vi "OpenDBEditor.vi"   [LabVIEW 2021]
types:
  T1 = enum32{"Invalid", "Standard", "Closed", "Hidden", "Minimized", "Maximized"}
  T2 = typedef "ConfigurationData.ctl" = cluster{"DataSetFilePath":path, "DefaultErrorCreationType":string, "StartOfErrorRange":i32, "EndOfErrorRange":i32}
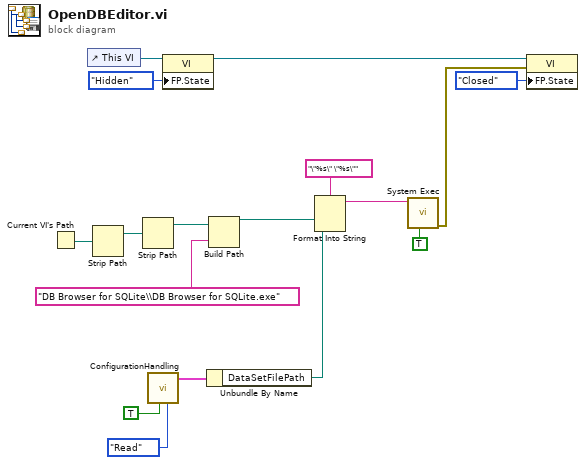
[diagram p0: block diagram]
diagram:
  n1 = Current VI's Path() -> (path=w16:path)
  n2 = control-ref of="This VI"() -> (w4:refnum<vi>)
  n3 = Strip Path(path=w16) -> (stripped path=w15:path)  [unwired: 1 out]
  n4 = Strip Path(path=w15) -> (stripped path=w14:path)  [unwired: 1 out]
  n5 = call "ConfigurationHandling.vi"("Function"=enum16{"Read", "Write"}."Read", "ForceReload"=TRUE) -> ("SettingsOut"=w8:T2)  [unwired: 9 in]
  n6 = property class="VI"(reference=w4, "FP.State"=T1."Hidden" ("Front Panel Window:State")) -> (reference out=w2:refnum<vi>)  [unwired: 1 in, 1 out]
  n7 = Unbundle By Name(w8) -> ("DataSetFilePath"=w7:path)
  n8 = Build Path(base path=w14, name or relative path="DB Browser for SQLite\\DB Browser for SQLite.exe") -> (appended path=w11:path)
  n9 = Format Into String(format string="\"%s\" \"%s\"" ("command line"), w11, w7) -> (resulting string=w6:string)  [unwired: 2 in, 1 out]
  n10 = call <vilib>:"System Exec.vi"("run minimized? (F)"=TRUE, "command line"=w6) -> ("error out"=w17:errorcluster)  [unwired: 6 in, 3 out]
  n11 = property class="VI"(reference=w2, error in=w17, "FP.State"=T1."Closed" ("Front Panel Window:State")) -> ()  [unwired: 2 out]
